vi "Next Step.vi"(8 "error in (no error)":errorcluster, 11 "Pulse Gen Basic Scan in":refnum<class "Pulse Gen Basic Scan.lvclass">) -> (0 "error out":errorcluster, 1 "Current Step":u32, 2 "Current Position":dbl, 3 "Pulse Gen Basic Scan out":refnum<class "Pulse Gen Basic Scan.lvclass">)   [LabVIEW 2012, in "Pulse Gen Basic Scan.lvclass"]
doc: "(Dynamic) Move to the next preconfigured step of this Scanner, and return the current position (actual, not intended) of this Scanner. Increment the step counter by one."
uses:
  Pulse Gen Basic Scan.lvclass
  Scanner/Scanner.lvclass
  Pulse Gen Basic Scan.lvclass/Pulse Gen Basic Scan.ctl
  Instruments/Utility Classes/Scannable/Scannable.lvclass
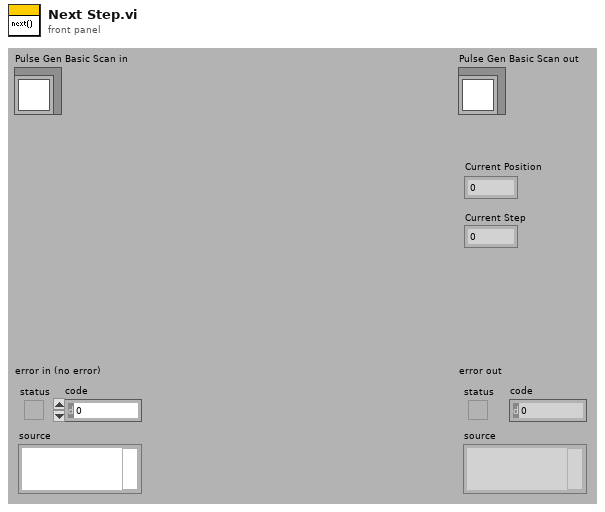
[diagram p1: front panel]
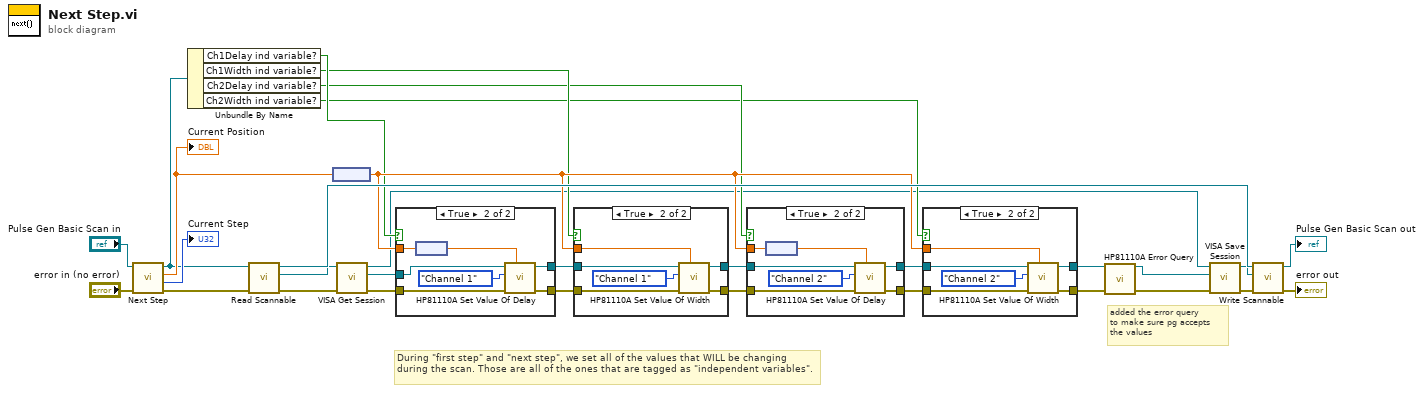
[diagram p0: block diagram]
diagram:
  # "added the error query\nto make sure pg accepts\nthe values"
  # "During \"first step\" and \"next step\", we set all of the values that WILL be changing during the scan. Those are all of the ones that are tagged as \"independent variables\"."
  n1 = call-parent "Next Step.vi"("error in (no error)"="error in (no error)", "Scanner in"="Pulse Gen Basic Scan in") -> ("error out"=w6:errorcluster, "Current Step"=→"Current Step":u32, "Current Position"=w10:dbl, "Scanner out"=w9:refnum<class "Pulse Gen Basic Scan.lvclass">)  [unwired: 6 in]
  "Current Position" <- w10
  n2 = Unbundle By Name(w9) -> ("Ch1Delay ind variable?"=w14:bool, "Ch1Width ind variable?"=w13:bool, "Ch2Delay ind variable?"=w12:bool, "Ch2Width ind variable?"=w11:bool)
  n3 = call-dynamic "Read Scannable.vi"("error in (no error)"=w6, "Scanner.lvclass in"=w9) -> ("error out"=w21:errorcluster, "Scannable.lvclass"=w19:refnum<class "Scannable.lvclass">, "Scanner.lvclass out"=w22:refnum<class "Pulse Gen Basic Scan.lvclass">)  [unwired: 7 out]
  n4 = node(w10) -> (w16:dbl[unit])
  n5 = call-dynamic "VISA Get Session.vi"("error in (no error)"=w21, "Instrument.lvclass in"=w19) -> ("error out"=w20:errorcluster, "VISA Resource Name"=w15:refnum<visa-resource-name>, "Instrument.lvclass out"=w5:refnum<class "Scannable.lvclass">)  [unwired: 7 out]
  n6 = case shown="True" w14 {
    tunnel: [w32 w40] -> w28
    tunnel: w20 -> [w33 w39]
    tunnel: [w33 w38] -> w25
    tunnel: w16 -> [_ w36]
    tunnel: w15 -> [w32 w34]
    frame False {
    }
    frame True {
      n7 = node(w36) -> (w35:dbl)
      n8 = call "HP81110A Set Value Of Delay.vi"("Delay Value (0.0)"=w35, "error in (no error)"=w39, "Channel (1:Channel 1)"=enum16{"Channel All ", "Channel 1", "Channel 2"}."Channel 1", "VISA session"=w34) -> ("error out"=w38:errorcluster, "dup VISA session"=w40:refnum<visa-resource-name>)  [unwired: 6 in]
    }
  }
  n9 = case shown="True" w13 {
    tunnel: w28 -> [w42 w48]
    tunnel: [w42 w47] -> w27
    tunnel: w25 -> [w41 w46]
    tunnel: [w41 w45] -> w24
    tunnel: w16 -> [_ w43]
    frame False {
    }
    frame True {
      n10 = call "HP81110A Set Value Of Width.vi"("Width Value (100.0E-9)"=w43, "error in (no error)"=w46, "Channel (1:Channel 1)"=enum16{"Channel All ", "Channel 1", "Channel 2"}."Channel 1", "VISA session"=w48) -> ("error out"=w45:errorcluster, "dup VISA session"=w47:refnum<visa-resource-name>)  [unwired: 6 in]
    }
  }
  n11 = case shown="True" w12 {
    tunnel: w27 -> [w50 w57]
    tunnel: [w50 w56] -> w26
    tunnel: w24 -> [w49 w55]
    tunnel: [w49 w54] -> w23
    tunnel: w16 -> [_ w52]
    frame False {
    }
    frame True {
      n12 = node(w52) -> (w51:dbl)
      n13 = call "HP81110A Set Value Of Delay.vi"("Delay Value (0.0)"=w51, "error in (no error)"=w55, "Channel (1:Channel 1)"=enum16{"Channel All ", "Channel 1", "Channel 2"}."Channel 2", "VISA session"=w57) -> ("error out"=w54:errorcluster, "dup VISA session"=w56:refnum<visa-resource-name>)  [unwired: 6 in]
    }
  }
  n14 = case shown="True" w11 {
    tunnel: w26 -> [w58 w65]
    tunnel: w23 -> [w59 w64]
    tunnel: [w59 w63] -> w3
    tunnel: w16 -> [_ w61]
    tunnel: [w58 w60] -> w4
    frame False {
    }
    frame True {
      n15 = call "HP81110A Set Value Of Width.vi"("Width Value (100.0E-9)"=w61, "error in (no error)"=w64, "Channel (1:Channel 1)"=enum16{"Channel All ", "Channel 1", "Channel 2"}."Channel 2", "VISA session"=w65) -> ("error out"=w63:errorcluster, "dup VISA session"=w60:refnum<visa-resource-name>)  [unwired: 6 in]
    }
  }
  n16 = call "HP81110A Error Query.vi"("VISA session"=w4, "error in (no error)"=w3) -> ("dup VISA session"=w2:refnum<visa-resource-name>, "error out"=w1:errorcluster)  [unwired: 10 in, 2 out]
  n17 = call-dynamic "VISA Save Session.vi"("error in (no error)"=w1, "VISA Resource Name"=w2, "Instrument.lvclass in"=w5) -> ("error out"=w17:errorcluster, "Instrument.lvclass out"=w18:refnum<class "Scannable.lvclass">)  [unwired: 7 out]
  n18 = call-dynamic "Write Scannable.vi"("error in (no error)"=w17, "Scannable.lvclass"=w18, "Scanner.lvclass in"=w22) -> ("error out"=→"error out":errorcluster, "Scanner.lvclass out"=→"Pulse Gen Basic Scan out":refnum<class "Pulse Gen Basic Scan.lvclass">)  [unwired: 7 out]
